vi "dl950 Test.vi"() -> ()   [LabVIEW 2019]
uses:
  <instrlib>/Yokogawa DL950 Series/Public/Data/Read Waveform (Single).vi
  <instrlib>/Yokogawa DL950 Series/Yokogawa DL950 Series.lvlib
panel:
  in  "Count (0: Infinity)":u32
  in  "Acquisition Mode (0: Normal)":i32(ring) items=["Normal", "Average", "Envelope"]
  in  "Record Length (0: 10k)":i32(ring) items=["10k", "25k", "50k", "100k", "250k", "500k", "1M", "2.5M", "5M", "10M", "25M", "50M", "100M", "250M", "500M", "1G", "2G", "4G", "5G", "10G", "20G", "50G"]
  in  "Source (1: CH1)":u16(ring)=1 items=["", "CH1", "CH2", "CH3", "CH4", "CH5", "CH6", "CH7", "CH8", "CH9", "CH10", "CH11", "CH12", "CH13", "CH14", "CH15", "CH16", "MATH1", "MATH2", "MATH3", "MATH4", "MATH5", "MATH6", "MATH7", "MATH8", "EVENT"]
  in  "Sub Channel (0: None)":i16(ring) items=["None", "SCH1", "SCH2", "SCH3", "SCH4", "SCH5", "SCH6", "SCH7", "SCH8", "SCH9", "SCH10", "SCH11", "SCH12", "SCH13", "SCH14", "SCH15", "SCH16", "SCH17", "SCH18", "SCH19", "SCH20", "SCH21", "SCH22", "SCH23", "SCH24", "SCH25", "SCH26", "SCH27", "SCH28", "SCH29", "SCH30", "SCH31", "SCH32", "SCH33", "SCH34", "SCH35", "SCH36", "SCH37", "SCH38", "SCH39", "SCH40", "SCH41", "SCH42", "SCH43", "SCH44", "SCH45", "SCH46", "SCH47", "SCH48", "SCH49", "SCH50", "SCH51", "SCH52", "SCH53", "SCH54", "SCH55", "SCH56", "SCH57", "SCH58", "SCH59", "SCH60", "SCH61", "SCH62", "SCH63", "SCH64"]
  in  "Timeout (10000 ms)":u32=10000
  out "Waveform Graph":waveform(dbl)(graph)
  in  "stop":bool
  in  "Enable Inverted Display (F: Off)":bool caption="Inverted Display (F: OFF)"
  in  "Bandwidth (0: Full)":i32(ring) items=["Full", "Auto", "0.1Hz", "1Hz", "2Hz", "8Hz", "30Hz", "40Hz", "400Hz", "500Hz", "4kHz", "5kHz", "10kHz", "20kHz", "40kHz", "50kHz", "80kHz", "160kHz", "320kHz", "400kHz", "500kHz", "640kHz", "1.28MHz", "2MHz", "2.56MHz", "5MHz"]
  in  "Probe Attenuation (3: 10:1)":i32(ring)=3 caption="Probe (10: 1)" items=["1:1", "2:1", "5:1", "10:1", "20:1", "50:1", "100:1", "200:1", "500:1", "1000:1", "2000:1", "5000:1", "10k:1", "20k:1", "50k:1", "0.1A:1V", "0.2A:1V", "0.5A:1V", "1A:1V", "2A:1V", "5A:1V", "10A:1V", "20A:1V", "50A:1V", "100A:1V", "200A:1V", "250A:1V", "400A:1V", "500A:1V", "1kA:1V", "2kA:1V", "5kA:1V", "10kA:1V", "20kA:1V", "50kA:1V", "NoSet"]
  in  "Vertical Coupling (1: DC)":i32(ring)=1 items=["AC", "DC", "Ground", "AC-RMS", "DC-RMS"]
  in  "Vertical Division (20: 50)":i32(ring)=20 items=["0.1m", "0.2m", "0.5m", "1m", "2m", "5m", "10m", "20m", "50m", "100m", "200m", "500m", "1", "2", "4", "5", "8", "10", "20", "40", "50", "80", "100", "200", "400", "500", "800", "1k", "2k", "4k", "5k", "8k", "10k", "20k", "25k", "50k", "100k", "250k", "500k", "1000k"]
  in  "Channel (1: CH1)":u16(ring)=1 items=["", "CH1", "CH2", "CH3", "CH4", "CH5", "CH6", "CH7", "CH8", "CH9", "CH10", "CH11", "CH12", "CH13", "CH14", "CH15", "CH16"]
  in  "Time Division (12: 1ms)":i32(ring)=12 items=["100ns", "200ns", "500ns", "1us", "2us", "5us", "10us", "20us", "50us", "100us", "200us", "500us", "1ms", "2ms", "5ms", "10ms", "20ms", "50ms", "100ms", "200ms", "500ms", "1s", "2s", "3s", "4s", "5s", "6s", "10s", "20s", "30s", "1min", "2min", "3min", "4min", "5min", "6min", "10min", "12min", "30min", "1hour", "2hour", "3hour", "4hour", "5hour", "6hour", "8hour", "10hour", "12hour", "1day", "2day", "3day", "4day", "5day"]
  out "read buffer":string
  out "error out":errorcluster
  in  "VISA resource name":refnum<visa-resource-name>
  in  "ID Query (True)":bool=TRUE
  in  "error in (no error)":errorcluster
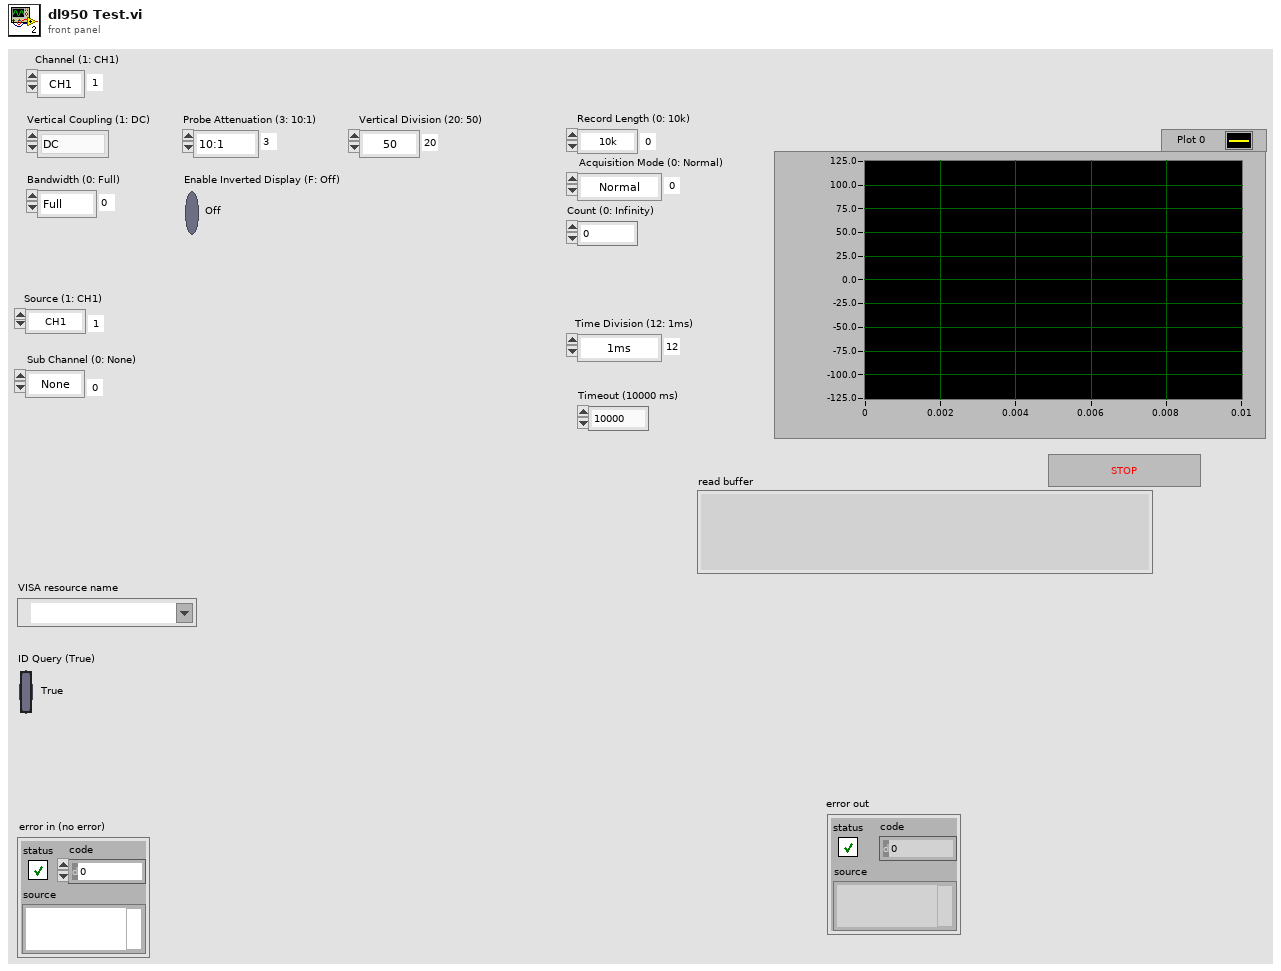
[diagram p1: front panel]
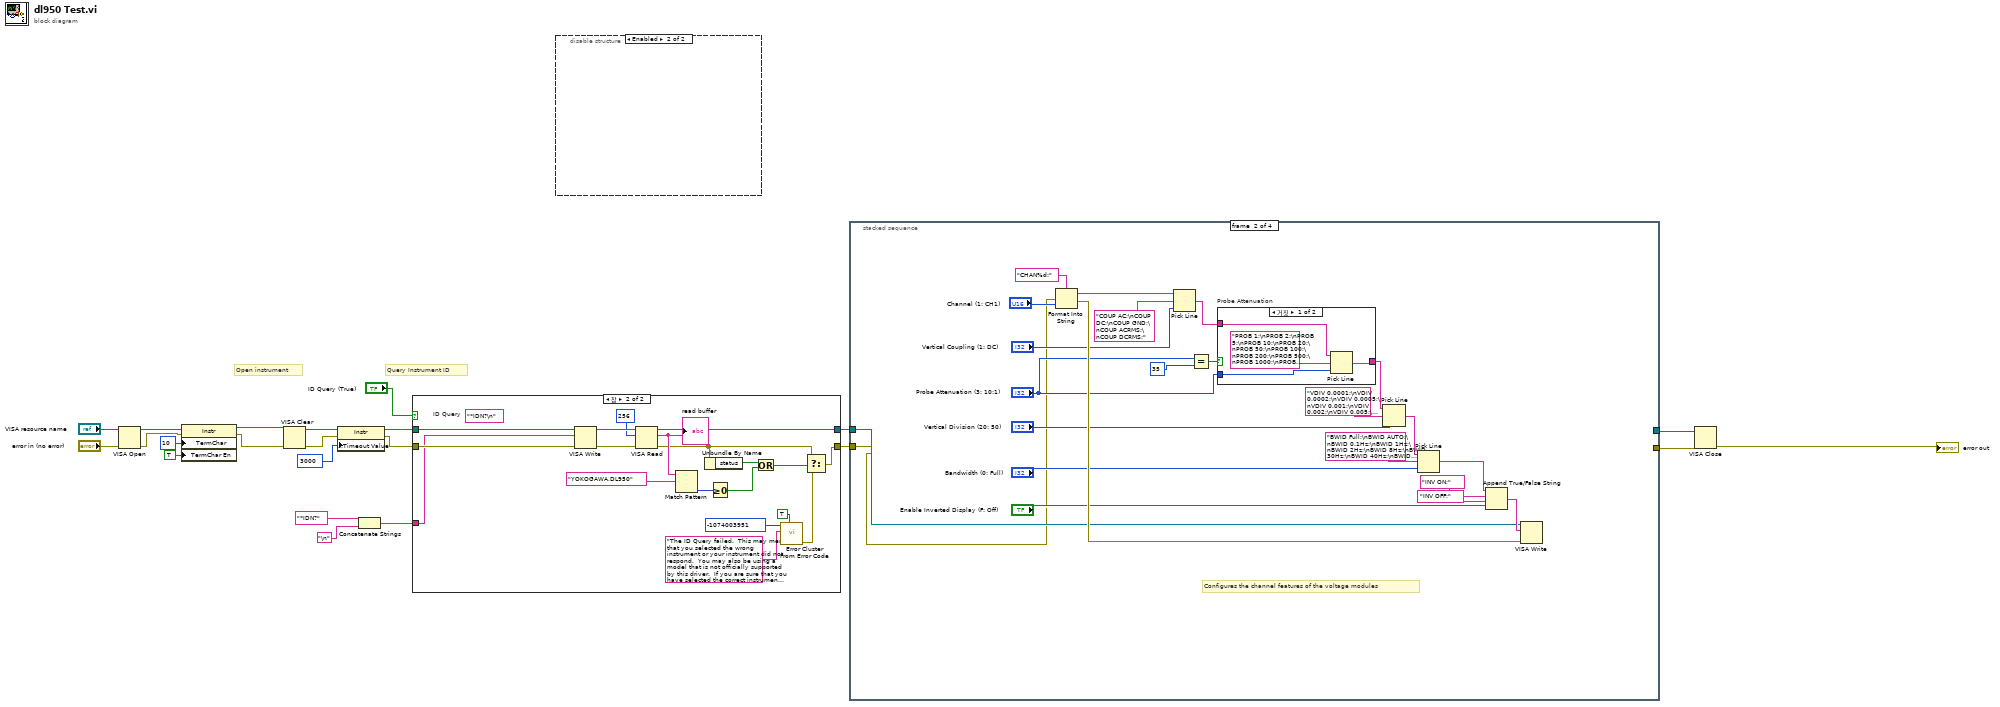
[diagram p0: block diagram]
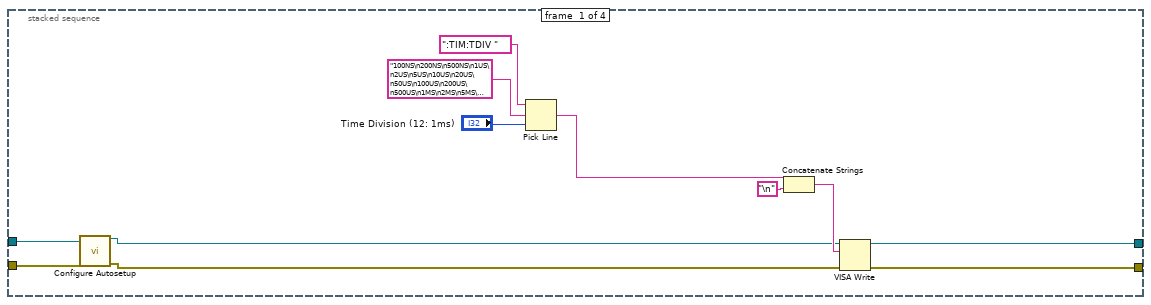
[diagram p2: hidden frame]
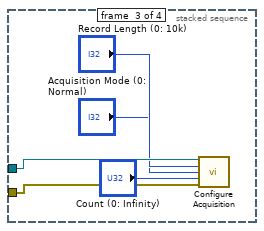
[diagram p4: hidden frame]
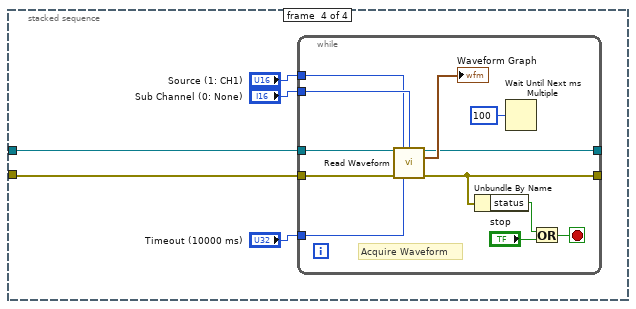
[diagram p5: hidden frame]
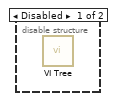
[diagram p6: hidden frame]
diagram:
  # "Query Instrument ID"
  # "Open instrument"
  n1 = VISA Open ("VISAオープン")(error in (no error)="error in (no error)", VISA resource name="VISA resource name") -> (VISA resource name=w9:refnum<visa-resource-name>, error out=w8:errorcluster)  [unwired: 3 in]
  n2 = property class="Instr"(reference=w9, error in=w8, "TermChar"=u8 10 ("Message Based Settings:Termination Character"), "TermChar En"=TRUE ("Message Based Settings:Termination Character Enable")) -> (reference out=w7:refnum<visa-resource-name>, error out=w6:errorcluster)
  n3 = VISA Clear ("VISAクリア")(VISA resource name=w7, error in (no error)=w6) -> (VISA resource name out=w18:refnum<visa-resource-name>, error out=w17:errorcluster)
  n4 = property on="プロパティノード" class="Instr"(reference=w18, error in=w17, "General Settings:Timeout Value"=u32 3000) -> (reference out=w16:refnum<visa-resource-name>, error out=w15:errorcluster)
  n5 = Concatenate Strings("*IDN?" ("Command"), "\n") -> (w12:string)
  n6 = case "ケースストラクチャ" shown="참" "ID Query (True)" {
    tunnel: [w23 w43] -> w1
    tunnel: [w24 w40] -> w2
    tunnel: w16 -> [w24 w41]
    tunnel: w15 -> [w23 w42]
    tunnel: w12 -> [_ w25]
    frame False {
    }
    frame True {
      (unwired) "*IDN?\n"  # ID Query
      n7 = VISA Write ("VISA書き込み")(VISA resource name=w41, write buffer=w25, error in (no error)=w42) -> (VISA resource name out=w28:refnum<visa-resource-name>, error out=w27:errorcluster)  [unwired: 1 out]
      n8 = VISA Read ("VISA読み取り")(VISA resource name=w28, byte count=u32 256, error in (no error)=w27) -> (VISA resource name out=w40:refnum<visa-resource-name>, read buffer=w39:string, error out=w32:errorcluster)  [unwired: 1 out]
      "read buffer" <- w39
      n9 = Match Pattern ("パターンで一致")(string=w39, regular expression="YOKOGAWA,DL950") -> (offset past match=w33:i32)  [unwired: 1 in, 3 out]
      n10 = Unbundle By Name ("名前でバンドル解除")(w32) -> ("status"=w30:bool)
      n11 = Greater Or Equal To 0? ("0Èã?")(x=w33) -> (x >= 0?=w29:bool)
      n12 = Or(x=w30, y=w29) -> (x .or. y?=w31:bool)
      n13 = call <vilib>:"Error Cluster From Error Code.vi"("show call chain? (False)"=TRUE, "error message (\"\")"="The ID Query failed.  This may mean that you selected the wrong instrument or your instrument did not respond.  You may also be using a model that is not officially supported by this driver.  If you are sure that you have selected the correct instrument and it is responding, try disabling the ID Query." ("Source (VI Name)"), "error code (0)"=-1074003951 ("Code")) -> ("error out"=w37:errorcluster)  [unwired: 6 in]
      n14 = Select ("‘I‘ð")(t=w32, s=w31, f=w37) -> (s? t:f=w43:errorcluster)
    }
  }
  n15 = disable-structure shown="Enabled" {
    frame Disabled {
      n16 = call <instrlib>:"VI Tree.vi"() -> ()  [unwired: 12 in]
    }
    frame Enabled {
    }
  }
  n17 = stacked-sequence {
    tunnel: [w52 _ _ _] -> w4
    tunnel: [w51 _ _ _] -> w3
    tunnel: w2 -> [w47 w57 w88 w93]
    tunnel: w1 -> [w45 w56 w87 w92]
    frame #0 {
      n18 = call <instrlib>:"Configure Autosetup.vi"("VISA resource name"=w47, "error in (no error)"=w45) -> ("VISA resource name out"=w46:refnum<visa-resource-name>, "error out"=w44:errorcluster)  [unwired: 12 in]
      n19 = Pick Line ("ライン選択")(string ("")=":TIM:TDIV ", multi-line string="100NS\n200NS\n500NS\n1US\n2US\n5US\n10US\n20US\n50US\n100US\n200US\n500US\n1MS\n2MS\n5MS\n10MS\n20MS\n50MS\n100MS\n200MS\n500MS\n1S\n2S\n3S\n4S\n5S\n6S\n10S\n20S\n30S\n60S\n120S\n180S\n240S\n300S\n360S\n600S\n720S\n1800S\nHOUR1\nHOUR2\nHOUR3\nHOUR4\nHOUR5\nHOUR6\nHOUR8\nHOUR10\nHOUR12\nDAY1\nDAY2\nDAY3\nDAY4\nDAY5", line index="Time Division (12: 1ms)") -> (output string=w49:string)
      n20 = Concatenate Strings(w49, "\n") -> (w48:string)
      n21 = VISA Write ("VISA書き込み")(VISA resource name=w46, write buffer=w48, error in (no error)=w44) -> (VISA resource name out=w52:refnum<visa-resource-name>, error out=w51:errorcluster)  [unwired: 1 out]
    }
    frame #1 {
      # "Configures the channel features of the voltage modules"
      n22 = Format Into String ("文字列にフォーマット")(format string="CHAN%d:", error in=w56, "Channel (1: CH1)") -> (resulting string=w70:string, error out=w78:errorcluster)  [unwired: 1 in]
      n23 = Pick Line ("ライン選択")(string ("")=w70, multi-line string="COUP AC;\nCOUP DC;\nCOUP GND;\nCOUP ACRMS;\nCOUP DCRMS;", line index="Vertical Coupling (1: DC)") -> (output string=w71:string)
      n24 = Equal?(x="Probe Attenuation (3: 10:1)", y=35) -> (x = y?=w76:bool)
      n25 = case "Probe Attenuation" shown="거짓" w76 {
        tunnel: "Probe Attenuation (3: 10:1)" -> [w79 _]
        tunnel: w71 -> [w81 w83]
        tunnel: [w80 w83] -> w72
        frame False {
          n26 = Pick Line ("ライン選択")(string ("")=w81, multi-line string="PROB 1;\nPROB 2;\nPROB 5;\nPROB 10;\nPROB 20;\nPROB 50;\nPROB 100;\nPROB 200;\nPROB 500;\nPROB 1000;\nPROB 2000;\nPROB 5000;\nPROB 10000;\nPROB 20000;\nPROB 50000;\nPROB C0_1;\nPROB C0_2;\nPROB C0_5;\nPROB C1;\nPROB C2;\nPROB C5;\nPROB C10;\nPROB C20;\nPROB C50;\nPROB C100;\nPROB C200;\nPROB C250;\nPROB C400;\nPROB C500;\nPROB C1000;\nPROB C2000;\nPROB C5000;\nPROB C10000;\nPROB C20000;\nPROB C50000;", line index=w79) -> (output string=w80:string)
        }
        frame True {
        }
      }
      n27 = Pick Line ("ライン選択")(string ("")=w72, multi-line string="VDIV 0.0001;\nVDIV 0.0002;\nVDIV 0.0005;\nVDIV 0.001;\nVDIV 0.002;\nVDIV 0.005;\nVDIV 0.01;\nVDIV 0.02;\nVDIV 0.05;\nVDIV 0.1;\nVDIV 0.2;\nVDIV 0.5;\nVDIV 1;\nVDIV 2;\nVDIV 4;\nVDIV 5;\nVDIV 8;\nVDIV 10;\nVDIV 20;\nVDIV 40;\nVDIV 50;\nVDIV 80;\nVDIV 100;\nVDIV 200;\nVDIV 400;\nVDIV 500;\nVDIV 800;\nVDIV 1000;\nVDIV 2000;\nVDIV 4000;\nVDIV 5000;\nVDIV 8000;\nVDIV 10000;\nVDIV 20000;\nVDIV 25000;\nVDIV 50000;\nVDIV 100000;\nVDIV 250000;\nVDIV 500000;\nVDIV 1000000;", line index="Vertical Division (20: 50)") -> (output string=w73:string)
      n28 = Pick Line ("ライン選択")(string ("")=w73, multi-line string="BWID Full;\nBWID AUTO;\nBWID 0.1Hz;\nBWID 1Hz;\nBWID 2Hz;\nBWID 8Hz;\nBWID 30Hz;\nBWID 40Hz;\nBWID 400Hz;\nBWID 500Hz;\nBWID 4kHz;\nBWID 5kHz;\nBWID 10kHz;\nBWID 20kHz;\nBWID 40kHz;\nBWID 50kHz;\nBWID 80kHz;\nBWID 160kHz;\nBWID 320kHz;\nBWID 400KHz;\nBWID 500kHz;\nBWID 640kHz;\nBWID 1.28MHz;\nBWID 2MHz;\nBWID 2.56MHz;\nBWID 5MHz;\n", line index="Bandwidth (0: Full)") -> (output string=w77:string)
      n29 = Append True/False String ("True/False 文字列を追加")(1:"Enable Inverted Display (F: Off)", 2:"INV OFF;", 3:"INV ON;", 4:w77) -> (0:w69:string)
      n30 = VISA Write ("VISA書き込み")(VISA resource name=w57, write buffer=w69, error in (no error)=w78) -> ()  [unwired: 3 out]
    }
    frame #2 {
      n31 = call <instrlib>:"Configure Acquisition.vi"("VISA resource name"=w88, "Record Length (0: 10k)"="Record Length (0: 10k)", "Acquisition Mode (0: Normal)"="Acquisition Mode (0: Normal)", "Count (0: Infinity)"="Count (0: Infinity)", "error in (no error)"=w87) -> ()  [unwired: 9 in, 2 out]
    }
    frame #3 {
      n32 = while "Whileループ" {
        tunnel: [w99] -> _
        tunnel: [w104] -> _
        tunnel: w92 -> [w97]
        tunnel: w93 -> [w103]
        tunnel: "Timeout (10000 ms)" -> [w96]
        tunnel: "Sub Channel (0: None)" -> [w95]
        tunnel: "Source (1: CH1)" -> [w94]
        stop <- w100 stop-if-true
        # "Acquire Waveform"
        n33 = call-poly <instrlib>:"Read Waveform.vi"("VISA resource name"=w103, "Source (1: CH1)"=w94, "Sub Channel (0 :None)"=w95, "error in (no error)"=w97, "Timeout (10000 ms)"=w96) -> ("VISA resource name out"=w104:refnum<visa-resource-name>, "Waveform Data"=→"Waveform Graph":waveform(dbl), "error out"=w99:errorcluster)  [unwired: 8 in]
        n34 = Unbundle By Name ("名前でバンドル解除")(w99) -> ("status"=w101:bool)
        n35 = Wait Until Next ms Multiple ("次のミリ秒倍数まで待機")(millisecond multiple=u32 100) -> ()  [unwired: 1 out]
        n36 = Or(x=w101, y="stop") -> (x .or. y?=w100:bool)
      }
    }
  }
  n37 = VISA Close(VISA resource name=w4, error in (no error)=w3) -> (error out=→"error out":errorcluster)
